vi "read_ini.vi"(8 "error in (no error)":errorcluster caption="错误输入（无错误）", 9 "section name":string, 10 "file ref in":T1, 11 "MotorSystem 输入":refnum<class "MotorSystem.lvclass">) -> (0 "error out":errorcluster caption="错误输出", 2 "file ref out":T1, 3 "MotorSystem 输出":refnum<class "MotorSystem.lvclass">)   [LabVIEW 2016, in "MotionControl_UFO_3DOF.lvlib" / "MotorSystem.lvclass"]
uses:
  <userlib>/MotionControl_UFO_3DOF/MotorSystem/MotorSystem.lvclass
  <vilib>/Utility/config.llb/Config Data RefNum.ctl
  <userlib>/MotionControl_UFO_3DOF/MotorSystem/MotorSystem.lvclass/MotorSystem.ctl
  <userlib>/MotionControl_UFO_3DOF/MotorSystem/MotionCluster.ctl
  <userlib>/MotionControl_UFO_3DOF/OneMotion/OneMotion.lvclass
  <vilib>/Utility/config.llb/Read Key (String).vi
  <vilib>/Utility/config.llb/Read Key (I32).vi
  <vilib>/Utility/config.llb/Read Key (Boolean).vi
  <vilib>/ErrorRing/Error Ring.xnode
  <vilib>/Utility/config.llb/NI_LVConfig.lvlib
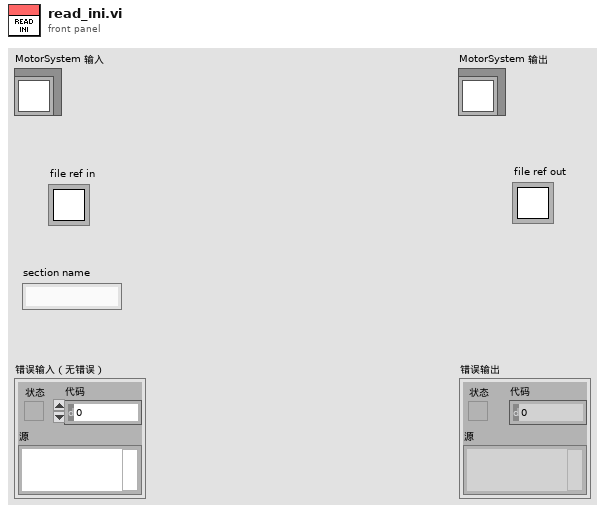
[diagram p1: front panel]
types:
  T1 = typedef "NI_LVConfig.lvlib/Config Data RefNum.ctl" = refnum<k1>
  T2 = typedef "MotionControl_UFO_3DOF.lvlib/StepMotor.lvclass/DEV_INFO.ctl" = cluster{"设备类型(0x01 = RS232CAN;0x02 = WIFI2RS232CAN;0x04 = USBCAN)":u32, "设备编号":u32, "系统为RS232CAN网关设备分配的COM口编号，这个成员变量只对\nRS232网关设备有用":u32, "RS232CAN网关设备与PC通讯的串口波特率，这个成员变量只对\nRS232网关设备有用":u32, "保存网关设备的名称":string}
  T3 = cluster{"complete dimension names":string[], "dimension names cluster ":cluster{"name 1":string, "name 2":string, "name 3":string}}
  T4 = typedef "MotionControl_UFO_3DOF.lvlib/MotorSystem.lvclass/MotionCluster.ctl" = cluster{"OneMotion.lvclass":refnum<class "OneMotion.lvclass">, "connected?":bool, "default enabled?":bool, "enabled?":bool}
  T5 = typedef "MotionControl_UFO_3DOF.lvlib/MotorSystem.lvclass/SavedPosCluster.ctl" = cluster{"name":string, "command list":T6}
  T6 = typedef "MotionControl_UFO_3DOF.lvlib/MotorSystem.lvclass/CommandList.ctl" = cluster{"cmd":T7, "cmd info":T8[]}[]
  T7 = typedef "MotionControl_UFO_3DOF.lvlib/MotorSystem.lvclass/cmd_system.ctl" = enum16{"NONE", "MOVE_SYSTEM", "WAIT_UNTIL_MOVE_DONE", "EXIT", "WAIT_UNTIL_SELECTED_MOVE_DONE", "WAIT_A_TIME"}
  T8 = typedef "MotionControl_UFO_3DOF.lvlib/MotorSystem.lvclass/SavedDimensionCluster.ctl" = cluster{"dimension name":string, "pos":dbl, "unit mode":T9, "unit conversion ratio":dbl}
  T9 = typedef "MotionControl_UFO_3DOF.lvlib/OneMotion.lvclass/unit mode.ctl" = enum16{"motor (pulse)", "linear (mm) or radial (degree)"}
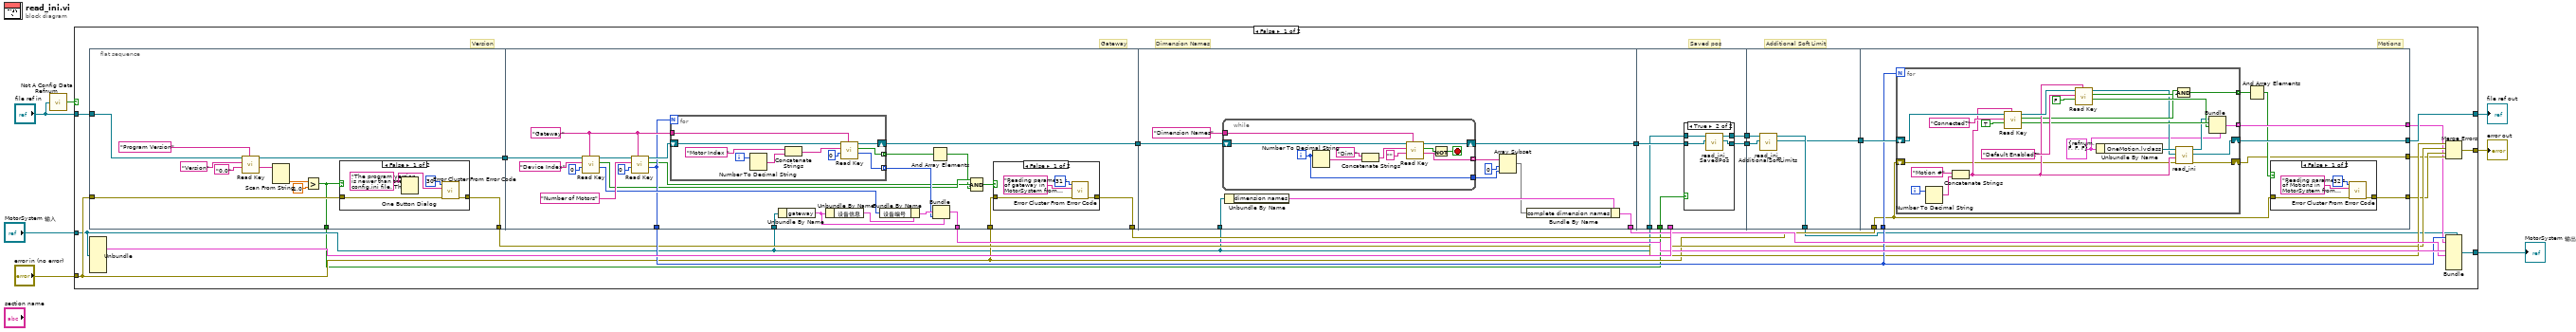
[diagram p0: block diagram]
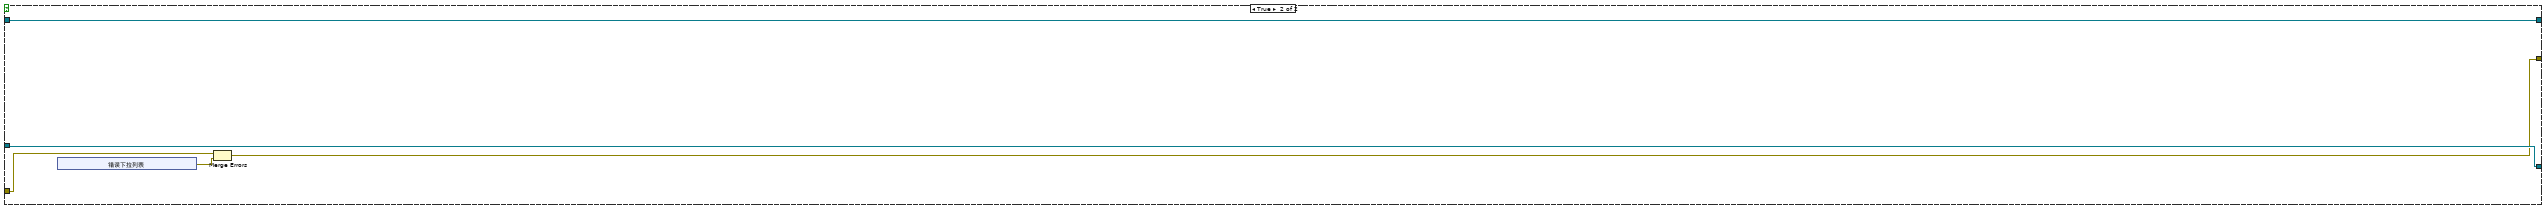
[diagram p6: hidden frame]
diagram:
  n1 = call <vilib>:"Not A Config Data Refnum.vi"("refnum"="file ref in") -> ("not a config data refnum"=w4:bool)
  n2 = case shown="False" w4 {
    tunnel: [w15 w160] -> w7
    tunnel: [w21 w163] -> w5
    tunnel: "MotorSystem 输入" -> [w13 w163]
    tunnel: "error in (no error)" -> [w18 w161]
    tunnel: "file ref in" -> [w30 w159]
    tunnel: [w25 w159] -> w1
    frame False {
      # "Additional Soft Limit"
      # "Saved pos"
      # "Dimension Names"
      # "Version"
      # "Motions"
      # "Gateway"
      n3 = flat-sequence {
        tunnel: w30 -> [w41]
        tunnel: [w40] -> w29
        tunnel: w18 -> [w36]
        tunnel: [w34] -> w20
        tunnel: [w31] -> w8
        tunnel: [w64] -> w28
        tunnel: w29 -> [w69]
        tunnel: w13 -> [w62]
        tunnel: [w56] -> w22
        tunnel: [w54] -> w24
        tunnel: w18 -> [w48]
        tunnel: [w47] -> w19
        tunnel: w28 -> [w95]
        tunnel: [w94] -> w27
        tunnel: w13 -> [w92]
        tunnel: [w90] -> w23
        tunnel: w27 -> [w111]
        tunnel: [w109] -> w12
        tunnel: w26 -> [_]
        tunnel: w13 -> [w110]
        tunnel: [w108] -> w10
        tunnel: w8 -> [w107]
        tunnel: w12 -> [w119]
        tunnel: [w118] -> w11
        tunnel: w10 -> [w121]
        tunnel: [w120] -> w9
        tunnel: [w129] -> w25
        tunnel: w11 -> [w130]
        tunnel: w22 -> [w128]
        tunnel: [w127] -> w14
        tunnel: w18 -> [w123]
        tunnel: [w124] -> w17
        tunnel: [w122] -> w16
        frame #0 {
          n4 = call-poly <vilib>:"Read Key.vi"("section"="Program Version", "default value"="0.0", "key"="Version", "refnum"=w41) -> ("value"=w35:string, "refnum out"=w40:T1)  [unwired: 4 in, 2 out]
          n5 = Scan From String(input string=w35) -> (output 1=w33:dbl)  [unwired: 4 in, 3 out]
          n6 = Greater?(x=w33, y=1.0) -> (0:w31:bool)
          n7 = case shown="False" w31 {
            tunnel: w36 -> [w44 w46]
            tunnel: [w43 w46] -> w34
            frame False {
              w42 = "The program version is newer than the config.ini file. There was a change in saving the config file. Thereby the macros are not loaded here." ("error message (\"\")")
              n8 = One Button Dialog(message=w42) -> ()  [unwired: 1 in, 1 out]
              n9 = call <vilib>:"Error Cluster From Error Code.vi"("error in (no error)"=w44, "error message (\"\")"=w42, "error code (0)"=30) -> ("error out"=w43:errorcluster)  [unwired: 6 in]
            }
            frame True {
            }
          }
        }
        frame #1 {
          w66 = "Gateway"
          n10 = call-poly <vilib>:"Read Key.vi"("section"=w66, "default value"=0, "key"="Device Index", "refnum"=w69) -> ("value"=w59:i32, "found?"=w53:bool, "refnum out"=w68:T1)  [unwired: 4 in, 1 out]
          n11 = call-poly <vilib>:"Read Key.vi"("section"=w66, "default value"=0, "key"="Number of Motors", "refnum"=w68) -> ("value"=w56:i32, "found?"=w52:bool, "refnum out"=w65:T1)  [unwired: 4 in, 1 out]
          n12 = for {
            N: w56 -> [_]
            tunnel: w66 -> [w85]
            shift-right: [w83] -> w64
            shift-left: w65 -> [w84]
            tunnel: [w77] -> w55 mode=indexing
            tunnel: [w76] -> w51 mode=indexing
            i -> [w82]
            n13 = Number To Decimal String(number=w82) -> (decimal integer string=w80:string)  [unwired: 1 in]
            n14 = Concatenate Strings("Motor Index ", w80) -> (w79:string)
            n15 = call-poly <vilib>:"Read Key.vi"("section"=w85, "default value"=0, "key"=w79, "refnum"=w84) -> ("value"=w77:i32, "found?"=w76:bool, "refnum out"=w83:T1)  [unwired: 4 in, 1 out]
          }
          n16 = Unbundle By Name(w62) -> ("gateway"=w61:cluster{"CAN 波特率":u32, "设备信息":T2, "设备站点":u32[]})
          n17 = Unbundle By Name(w61) -> ("设备信息"=w60:T2)
          n18 = Bundle By Name(cluster=w60, "设备编号"=w59) -> (w58:T2)
          n19 = And Array Elements(Boolean array=w51) -> (logical AND=w50:bool)
          n20 = Bundle(cluster=w61, "设备信息"=w58, "设备站点"=w55) -> (w54:cluster{"CAN 波特率":u32, "设备信息":T2, "设备站点":u32[]})  [unwired: 1 in]
          n21 = Compound Arithmetic op=AND(w53, w52, w50) -> (w49:bool)
          n22 = case shown="False" w49 {
            tunnel: w48 -> [w72 w75]
            tunnel: [w71 w75] -> w47
            frame False {
              n23 = call <vilib>:"Error Cluster From Error Code.vi"("error in (no error)"=w72, "error message (\"\")"="Reading parameters of gateway in MotorSystem from file not found." ("error message (\"\")"), "error code (0)"=31) -> ("error out"=w71:errorcluster)  [unwired: 6 in]
            }
            frame True {
            }
          }
        }
        frame #2 {
          n24 = while {
            shift-right: [w105] -> w94
            shift-left: w95 -> [w106]
            tunnel: "Dimension Names" -> [w104]
            tunnel: [w99] -> w87 mode=indexing
            tunnel: [w96] -> w86
            i -> [w96]
            stop <- w97 stop-if-true
            n25 = Number To Decimal String(number=w96) -> (decimal integer string=w103:string)  [unwired: 1 in]
            n26 = Concatenate Strings("Dim ", w103) -> (w101:string)
            n27 = call-poly <vilib>:"Read Key.vi"("section"=w104, "default value"="", "key"=w101, "refnum"=w106) -> ("value"=w99:string, "found?"=w98:bool, "refnum out"=w105:T1)  [unwired: 4 in, 1 out]
            n28 = Not(x=w98) -> (.not. x?=w97:bool)
          }
          n29 = Unbundle By Name(w92) -> ("dimension names"=w91:T3)
          n30 = Array Subset(array=w87, index=0 ("索引"), length=w86) -> (w89:string[])
          n31 = Bundle By Name(cluster=w91, "complete dimension names"=w89) -> (w90:T3)
        }
        frame #3 {
          n32 = case shown="True" w107 {
            tunnel: w111 -> [w112 w117]
            tunnel: w110 -> [w113 w116]
            tunnel: [w112 w115] -> w109
            tunnel: [w113 w114] -> w108
            frame False {
            }
            frame True {
              n33 = call <userlib>:"read_ini_SavedPos.vi"("file ref in"=w117, "MotorSystem 输入"=w116) -> ("file ref out"=w115:T1, "MotorSystem 输出"=w114:refnum<class "MotorSystem.lvclass">)  [unwired: 7 in, 1 out]
            }
          }
        }
        frame #4 {
          n34 = call <userlib>:"read_ini_AdditionalSoftLimits.vi"("file ref in"=w119, "MotorSystem 输入"=w121) -> ("file ref out"=w118:T1, "MotorSystem 输出"=w120:refnum<class "MotorSystem.lvclass">)  [unwired: 7 in, 1 out]
        }
        frame #5 {
          n35 = for {
            N: w128 -> [_]
            shift-right: [w158] -> w129
            shift-left: w130 -> [w153]
            tunnel: [w144] -> w127 mode=indexing
            tunnel: [w140] -> w126 mode=indexing
            shift-right: [w138] -> w122
            shift-left: w123 -> [w139]
            i -> [w157]
            w136 = T4 {"OneMotion.lvclass"=refnum, "connected?"=FALSE, "default enabled?"=FALSE, "enabled?"=FALSE} ("簇")
            n36 = Number To Decimal String(number=w157) -> (decimal integer string=w156:string)  [unwired: 1 in]
            n37 = Concatenate Strings("Motion #", w156) -> (w150:string)
            n38 = call-poly <vilib>:"Read Key.vi"("section"=w150, "default value"=TRUE, "key"="Connected?", "refnum"=w153) -> ("value"=w148:bool, "found?"=w142:bool, "refnum out"=w152:T1)  [unwired: 4 in, 1 out]
            n39 = call-poly <vilib>:"Read Key.vi"("section"=w150, "default value"=FALSE, "key"="Default Enabled?", "refnum"=w152) -> ("value"=w146:bool, "found?"=w141:bool, "refnum out"=w137:T1)  [unwired: 4 in, 1 out]
            n40 = Unbundle By Name(w136) -> ("OneMotion.lvclass"=w143:refnum<class "OneMotion.lvclass">)
            n41 = call-dynamic "read_ini.vi"("error in (no error)"=w139, "section name"=w150, "file ref in"=w137, "OneMotion 输入"=w143) -> ("error out"=w138:errorcluster, "file ref out"=w158:T1, "OneMotion 输出"=w145:refnum<class "OneMotion.lvclass">)  [unwired: 5 in]
            n42 = Compound Arithmetic op=AND(w142, w141) -> (w140:bool)
            n43 = Bundle(cluster=w136, "OneMotion.lvclass"=w145, "connected?"=w148, "default enabled?"=w146) -> (w144:T4)  [unwired: 1 in]
          }
          n44 = And Array Elements(Boolean array=w126) -> (logical AND=w125:bool)
          n45 = case shown="False" w125 {
            tunnel: w123 -> [w132 w135]
            tunnel: [w131 w135] -> w124
            frame False {
              n46 = call <vilib>:"Error Cluster From Error Code.vi"("error in (no error)"=w132, "error message (\"\")"="Reading parameters of Motions in MotorSystem from file not found." ("error message (\"\")"), "error code (0)"=32) -> ("error out"=w131:errorcluster)  [unwired: 6 in]
            }
            frame True {
            }
          }
        }
      }
      n47 = Unbundle(w13) -> (w26:T5[])  [unwired: 7 out]
      n48 = Merge Errors(w20, w19, w17, w16) -> (w15:errorcluster)
      n49 = Bundle(cluster=w9, w22, w14, w24, w23) -> (w21:refnum<class "MotorSystem.lvclass">)  [unwired: 4 in]
    }
    frame True {
      n50 = xnode "错误下拉列表"() -> ("error out"=w162:errorcluster)
      n51 = Merge Errors(w161, w162) -> (w160:errorcluster)
    }
  }
  "error out" <- w7
  "MotorSystem 输出" <- w5
  "file ref out" <- w1
